vi "checkImageFolder.vi"(10 "Path":path) -> (2 "badPath":bool)   [LabVIEW 2014]
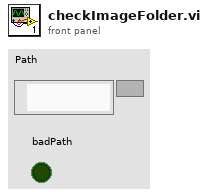
[diagram p1: front panel]
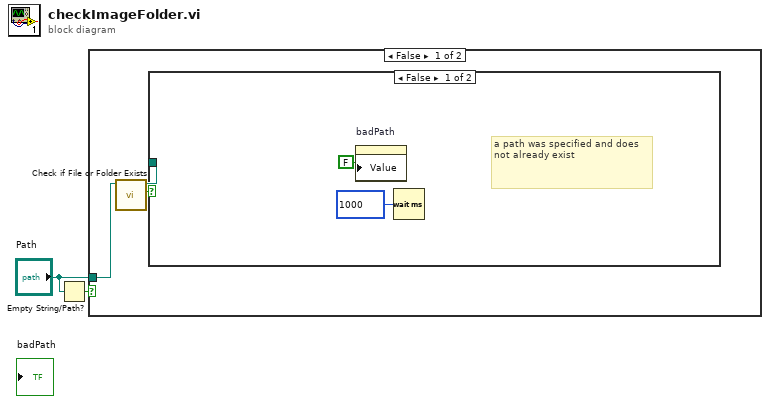
[diagram p0: block diagram]
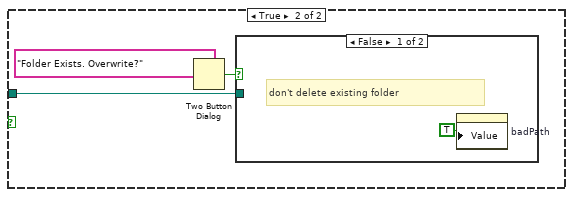
[diagram p2: hidden frame]
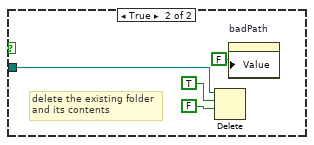
[diagram p3: hidden frame]
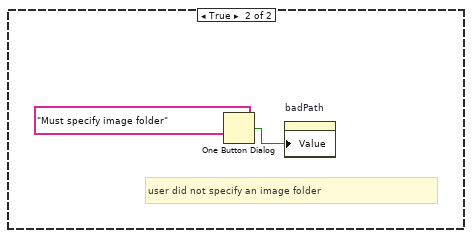
[diagram p4: hidden frame]
diagram:
  n1 = Empty String/Path?(string/path="Path") -> (empty?=w2:bool)
  n2 = case shown="False" w2 {
    tunnel: "Path" -> [w5 _]
    frame False {
      n3 = call <vilib>:"Check if File or Folder Exists.vi"("path"=w5) -> ("file or folder exists?"=w3:bool, "dup path"=w4:path)  [unwired: 8 in, 1 out]
      n4 = case shown="False" w3 {
        tunnel: w4 -> [_ w8]
        frame False {
          # "a path was specified and does not already exist"
          n5 = property on="badPath" class="Bool (strict)"("Value"=FALSE ("badPath")) -> ()  [unwired: 2 in, 2 out]
          n6 = Wait (ms)(milliseconds to wait=1000) -> ()  [unwired: 1 out]
        }
        frame True {
          n7 = Two Button Dialog(message="Folder Exists. Overwrite?") -> (T button?=w9:bool)  [unwired: 2 in]
          n8 = case shown="False" w9 {
            tunnel: w8 -> [_ w15]
            frame False {
              # "don't delete existing folder"
              n9 = property on="badPath" class="Bool (strict)"("Value"=TRUE ("badPath")) -> ()  [unwired: 2 in, 2 out]
            }
            frame True {
              # "delete the existing folder  and its contents"
              n10 = Delete(path (use dialog)=w15, entire hierarchy (F)=TRUE, confirm (F)=FALSE) -> ()  [unwired: 2 in, 3 out]
              n11 = property on="badPath" class="Bool (strict)"("Value"=FALSE ("badPath")) -> ()  [unwired: 2 in, 2 out]
            }
          }
        }
      }
    }
    frame True {
      # "user did not specify an image folder"
      n12 = One Button Dialog(message="Must specify image folder") -> (true=w17:bool)  [unwired: 1 in]
      n13 = property on="badPath" class="Bool (strict)"("Value"=w17) -> ()  [unwired: 2 in, 2 out]
    }
  }
